vi "Loop_RoboRio_SEN.vi"() -> ()   [LabVIEW 2017, in "System_Status.lvlib"]
uses:
  System_Status.lvlib
  _SHARE ALL/TypeDef Share All/CLUSTER_RoboRio_Status.ctl
  _SHARE ALL/TypeDef Share All/CLUSTER_RoboRio_Faults.ctl
  _SHARE ALL/TypeDef Share All/CLUSTER_RoboRio_Rails.ctl
  _SHARE ALL/TypeDef Share All/CLUSTER_RoboRio_SingleRail.ctl
  _SHARE ALL/Global Share All/Global_STOP.vi
  <vilib>/Rock Robotics/WPI/Power/WPI_Power Get 6Volt Rail Voltage and Current.vi
  <vilib>/Rock Robotics/WPI/Power/WPI_Power Get 5Volt Rail Voltage and Current.vi
  <vilib>/Rock Robotics/WPI/Power/WPI_Power Get 3Volt Rail Voltage and Current.vi
  Global_SEN Write_Data.vi
panel:
  out "Cycle Time (S)":dbl format="%.3g"
  in  "Target Time(ms)":u32=50
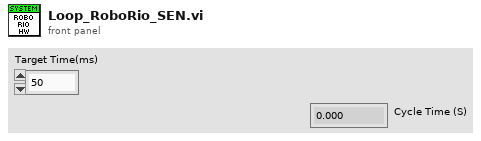
[diagram p1: front panel]
types:
  T1 = typedef "CLUSTER_RoboRio_Status.ctl" = cluster{"RoboRio Faults":T2, "RIO inpt vol (V)":dbl, "RIO inpt cur (A)":dbl, "RoboRio Rails":T3}
  T2 = typedef "CLUSTER_RoboRio_Faults.ctl" = cluster{"Inpt. V. Brn. Out":bool, "3.3V Usr Rail Shrt.":bool, "5 V Usr Rail Shrt.":bool, "6 V Usr. Rail Shrt.":bool, "5V Usr. Rail Brn. Out":bool}
  T3 = typedef "CLUSTER_RoboRio_Rails.ctl" = cluster{"3.3 Volt":T4, "5 Volt":T4, "6 Volt":T4}
  T4 = typedef "CLUSTER_RoboRio_SingleRail.ctl" = cluster{"Vol.  (V)":dbl, "Cur. (A)":dbl}
  T5 = cluster{"Target Time(ms)":u32, "Current Time":timestamp, "Previous Time":timestamp, "Cycle Time (S)":dbl, "RoboRio Status":T1}
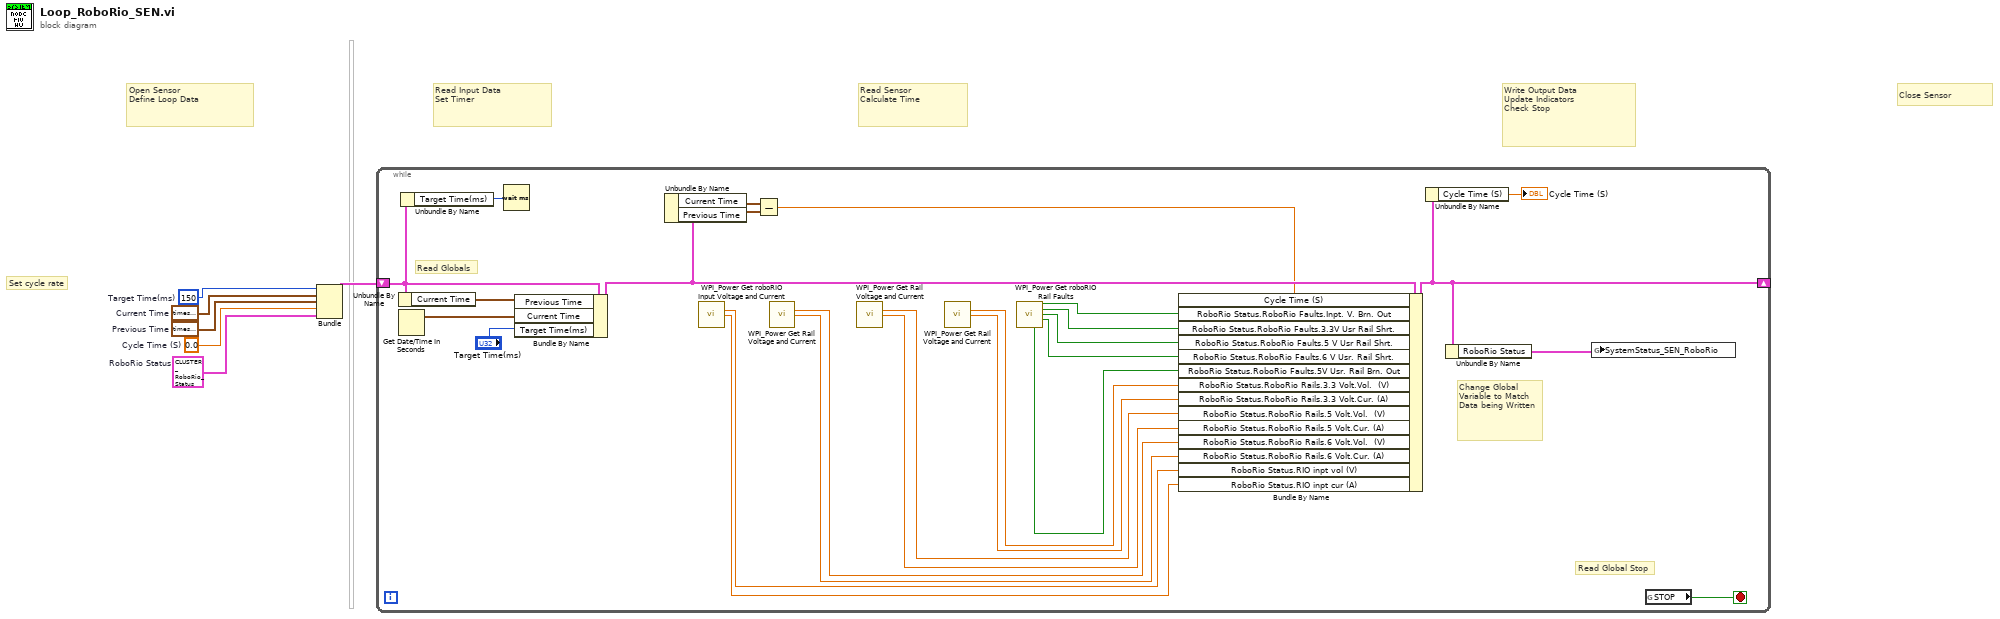
[diagram p0: block diagram]
diagram:
  w1 = T1 {"RoboRio Faults"={"Inpt. V. Brn. Out"=FALSE, "3.3V Usr Rail Shrt."=FALSE, "5 V Usr Rail Shrt."=FALSE, "6 V Usr. Rail Shrt."=FALSE, "5V Usr. Rail Brn. Out"=FALSE}, "RIO inpt vol (V)"=0.0, "RIO inpt cur (A)"=0.0, "RoboRio Rails"={"3.3 Volt"={"Vol.  (V)"=0.0, "Cur. (A)"=0.0}, "5 Volt"={"Vol.  (V)"=0.0, "Cur. (A)"=0.0}, "6 Volt"={"Vol.  (V)"=0.0, "Cur. (A)"=0.0}}}  # RoboRio Status
  w2 = 0.0  # Cycle Time (S)
  w6 = timestamp(0 s since 1904-01-01)  # Previous Time
  w5 = timestamp(0 s since 1904-01-01)  # Current Time
  w4 = u32 150  # Target Time(ms)
  # "Close Sensor"
  # "Write Output Data\nUpdate Indicators\nCheck Stop"
  # "Read Sensor\nCalculate Time"
  # "Read Input Data\nSet Timer"
  # "Open Sensor\nDefine Loop Data"
  # "Set cycle rate"
  n1 = Bundle("Target Time(ms)"=w4, "Current Time"=w5, "Previous Time"=w6, "Cycle Time (S)"=w2, "RoboRio Status"=w1) -> (w3:T5)  [unwired: 1 in]
  n2 = while {
    shift-right: [w22] -> _
    shift-left: w3 -> [w24]
    stop <- w32 stop-if-true
    # "Change Global\nVariable to Match\nData being Written"
    # "Read Globals"
    # "Read Global Stop"
    n3 = Unbundle By Name(w24) -> ("Current Time"=w29:timestamp)
    n4 = Get Date/Time In Seconds() -> (seconds since 1Jan1904=w30:timestamp)
    n5 = Unbundle By Name(w24) -> ("Target Time(ms)"=w23:u32)
    n6 = Wait (ms)(milliseconds to wait=w23) -> ()  [unwired: 1 out]
    n7 = Bundle By Name(cluster=w24, "Previous Time"=w29, "Current Time"=w30, "Target Time(ms)"="Target Time(ms)") -> (w25:T5)
    n8 = Unbundle By Name(w25) -> ("Current Time"=w28:timestamp, "Previous Time"=w27:timestamp)
    n9 = call <vilib>:"WPI_Power Get roboRIO Input Voltage and Current.vi"() -> ("roboRIO input voltage (V)"=w19:dbl, "roboRIO input current (A)"=w18:dbl)  [unwired: 13 in, 1 out]
    n10 = Subtract(x=w28, y=w27) -> (x-y=w20:dbl)
    n11 = call-poly <vilib>:"WPI_Power Get Rail Voltage and Current.vi"() -> ("6 volt rail voltage (V)"=w16:dbl, "6 volt rail current (A)"=w17:dbl)  [unwired: 13 in, 1 out]
    n12 = call-poly <vilib>:"WPI_Power Get Rail Voltage and Current.vi"() -> ("5 volt rail voltage (V)"=w14:dbl, "5 volt rail current (A)"=w15:dbl)  [unwired: 13 in, 1 out]
    n13 = call-poly <vilib>:"WPI_Power Get Rail Voltage and Current.vi"() -> ("3.3 volt rail voltage (V)"=w12:dbl, "3.3 volt rail current (A)"=w13:dbl)  [unwired: 13 in, 1 out]
    n14 = call <vilib>:"WPI_Power Get roboRIO Rail Faults.vi"() -> ("Input Voltage Brown Out"=w7:bool, "3.3V User Rail Short"=w8:bool, "5 V User Rail Short"=w9:bool, "6 V User Rail Short"=w10:bool, "5V User Rail Brown Out"=w11:bool)  [unwired: 10 in, 1 out]
    n15 = Bundle By Name(cluster=w25, "Cycle Time (S)"=w20, "RoboRio Status.RoboRio Faults.Inpt. V. Brn. Out"=w7, "RoboRio Status.RoboRio Faults.3.3V Usr Rail Shrt."=w8, "RoboRio Status.RoboRio Faults.5 V Usr Rail Shrt."=w9, "RoboRio Status.RoboRio Faults.6 V Usr. Rail Shrt."=w10, "RoboRio Status.RoboRio Faults.5V Usr. Rail Brn. Out"=w11, "RoboRio Status.RoboRio Rails.3.3 Volt.Vol.  (V)"=w12, "RoboRio Status.RoboRio Rails.3.3 Volt.Cur. (A)"=w13, "RoboRio Status.RoboRio Rails.5 Volt.Vol.  (V)"=w14, "RoboRio Status.RoboRio Rails.5 Volt.Cur. (A)"=w15, "RoboRio Status.RoboRio Rails.6 Volt.Vol.  (V)"=w16, "RoboRio Status.RoboRio Rails.6 Volt.Cur. (A)"=w17, "RoboRio Status.RIO inpt vol (V)"=w19, "RoboRio Status.RIO inpt cur (A)"=w18) -> (w22:T5)
    n16 = Unbundle By Name(w22) -> ("Cycle Time (S)"=→"Cycle Time (S)":dbl)
    n17 = Unbundle By Name(w22) -> ("RoboRio Status"=w31:T1)
    n18 = global write "Global_SEN Write_Data.vi" "SystemStatus_SEN_RoboRio"(w31) -> ()
    n19 = global read "Global_STOP.vi" "STOP"() -> (w32:bool)
  }
